vi "Post_Build.vi"(8 "error in (no error)":errorcluster, 9 "generated files":path[](array[path]), 11 "Build in":refnum<class "AB_Build.lvclass">) -> (0 "error out":errorcluster, 1 "GeneratedFiles":path[](array[path]), 3 "Build out":refnum<class "AB_Build.lvclass">)   [LabVIEW 2020, in "AB_Deployment.lvlib"]
uses:
  <vilib>/AppBuilder/AB_Classes/Deployment/AB_Deployment.lvlib
  <vilib>/AppBuilder/AB_Classes/Build/AB_Build.lvclass
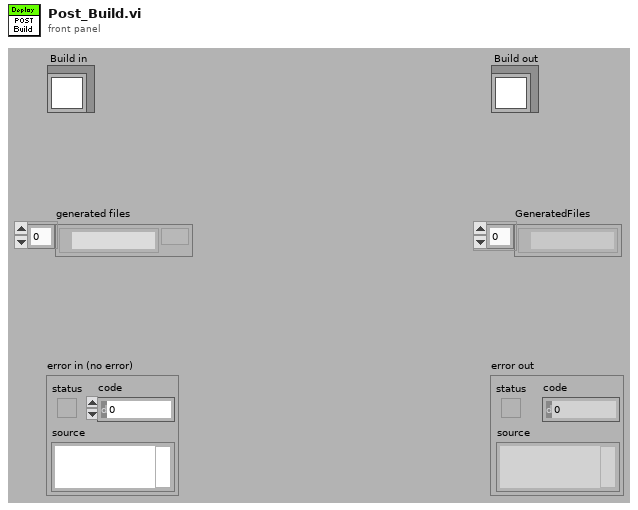
[diagram p1: front panel]
types:
  T1 = typedef "AB_Build.ctl" = cluster{"buildSpecName":string, "buildSpecDescription":string, "destinations":refnum<class "AB_Destination.lvclass">[], "exclusionOption":T2, "defaultLanguage":string, "supportedLanguages":string[], "excludedDirectories":path[], "buildContext":refnum<vi>, "buildObject":T3, "preview":bool, "programatic":bool, "progressBarEvents":T4, "userLog_Path":path, "preActionID":string, "preAction_Path":path, "postActionID":string, "postAction_Path":path, "eng_checkForBrokenVIs?":bool, "eng_verboseLinkerErrors?":bool, "localDest_Path":path, "targetDest_Path":path, "removeVIObject":u16, "cache":refnum<class "PreviewCache.lvclass">, "use cache":bool, "previewCache_ID":string, "buildCache_ID":string, "eng_TempLocalDest_Path":path, "eng_collectDependencies?":bool, "versionInfo":cluster{"buildVersion":cluster{"major":u16, "minor":u16, "patch":u16, "build":u16}, "autoIncrement":bool}, "eng_enableVIChecksums":bool}
  T2 = typedef "AB_Exclusion_Option.ctl" = cluster{"typedefs":bool, "polymorphicVIs":bool, "unusedLibraryItems":bool, "modifyLibraryFile":bool, "edit-timeDependencies":bool, "inlineVIs":bool, "dependent PPLs":bool, "dependent DLLs":bool}
  T3 = typedef "ItemRef.ctl" = u64
  T4 = typedef "provcom_ProgressBar_Events.ctl" = cluster{"newJob":refnum<user-event>, "newItem":refnum<user-event>, "errorMsg":T5, "cancel":refnum<user-event>}
  T5 = typedef "mxLvBuildError.ctl" = refnum<user-event>
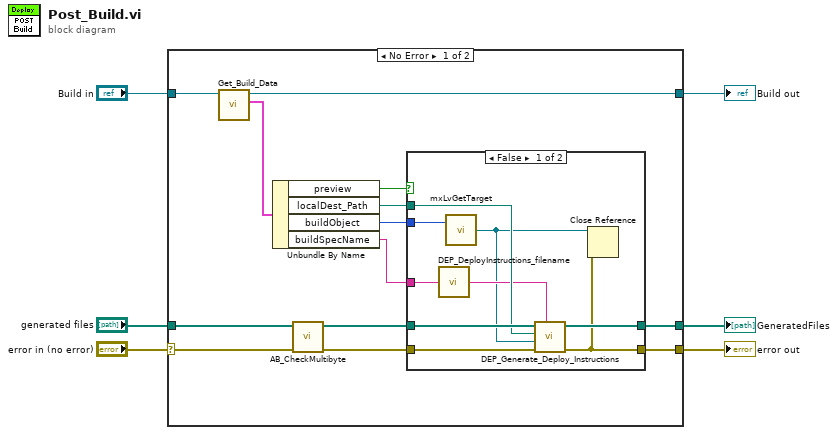
[diagram p0: block diagram]
diagram:
  n1 = case shown="No Error" "error in (no error)" {
    selector: "error in (no error)" -> [w17 w31]
    tunnel: [w16 w32] -> w6
    tunnel: "Build in" -> [w15 w32]
    tunnel: [w19 w31] -> w4
    tunnel: [w18 _] -> w3
    tunnel: "generated files" -> [w7 _]
    frame No Error {
      n2 = call <vilib>:"Get_Build_Data.vi"("Class in"=w15) -> ("data"=w14:T1, "Class out"=w16:refnum<class "AB_Build.lvclass">)  [unwired: 8 in, 1 out]
      n3 = Unbundle By Name(w14) -> ("preview"=w11:bool, "localDest_Path"=w13:path, "buildObject"=w12:T3, "buildSpecName"=w10:string)
      n4 = call <vilib>:"AB_CheckMultibyte.vi"("error in (no error)"=w17, "generated files"=w7) -> ("error out"=w8:errorcluster, "generated files out"=w9:path[])  [unwired: 8 in]
      n5 = case shown="False" w11 {
        tunnel: [w21 w29] -> w19
        tunnel: [w28 w30] -> w18
        tunnel: w8 -> [w27 w29]
        tunnel: w9 -> [w26 w30]
        tunnel: w13 -> [w25 _]
        tunnel: w12 -> [w24 _]
        tunnel: w10 -> [w20 _]
        frame False {
          n6 = call <resource>:"DEP_DeployInstructions_filename.vi"("prefix"=w20) -> ("deploy instructions filename"=w23:string)  [unwired: 4 in]
          n7 = call <resource>:"mxLvGetTarget.vi"("Item"=w24) -> ("Target"=w22:refnum<vi>)  [unwired: 1 in, 2 out]
          n8 = call <resource>:"DEP_Generate_Deploy_Instructions.vi"("deploy instructions filename"=w23, "error in (no error)"=w27, "TargetItem"=w22, "localDestPath"=w25, "Generated files"=w26) -> ("error out"=w21:errorcluster, "Generated files out"=w28:path[])  [unwired: 5 in]
          n9 = Close Reference(reference=w22, error in (no error)=w21) -> ()  [unwired: 1 out]
        }
        frame True {
        }
      }
    }
    frame Error {
    }
  }
  "error out" <- w4
  "GeneratedFiles" <- w3
  "Build out" <- w6
